vi "Teleop.vi"(10 "Match Info":T1={"Autonomous Elapsed Seconds"=0.0, "TeleOp Elapsed Seconds"=0.0, "Disabled Elapsed Seconds"=0.0, "Visited Autonomous"=FALSE, "Visited TeleOp"=FALSE, "Visited Disabled"=FALSE, "Autonomous Settings"={"Autonomous Style"=enum."Independent", "VI Refnum"=refnum}}, 11 "Call Context":T2) -> ()   [LabVIEW 2012]
doc: "This VI is called for each TeleOp packet received from the DS where the robot is not disabled. It is often used to read from the joysticks and update I/O or to update setpoints for timed control loops. It should complete and return within 20 milliseconds or it may miss DS packets."
uses:
  <vilib>/Rock Robotics/WPI/DriverStation/WPI_DriverStationDerivedRobotMode.ctl
  <vilib>/Rock Robotics/WPI/DriverStation/WPI_DriverStationMatch Info.ctl
  <vilib>/Rock Robotics/WPI/Relay/WPI_RelayValue.ctl
  Robot Global Data.vi
  <vilib>/Rock Robotics/WPI/Joystick/WPI_JoystickGetSetRefNum.vi
panel:
  in  "Ext Const":dbl=0.5
  in  "Dep Const":dbl=1.0
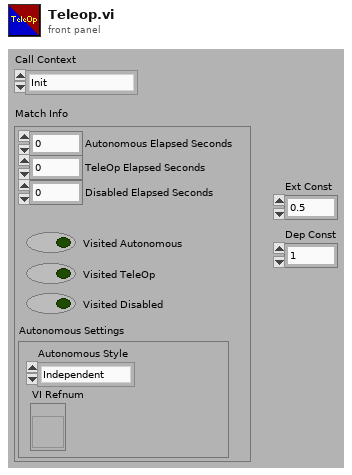
[diagram p1: front panel]
types:
  T1 = typedef "WPI_DriverStationMatch Info.ctl" = cluster{"Autonomous Elapsed Seconds":dbl, "TeleOp Elapsed Seconds":dbl, "Disabled Elapsed Seconds":dbl, "Visited Autonomous":bool, "Visited TeleOp":bool, "Visited Disabled":bool, "Autonomous Settings":cluster{"Autonomous Style":enum16{"Iterative", "Independent"}, "VI Refnum":refnum<vi>}}
  T2 = typedef "WPI_DriverStationDerivedRobotMode.ctl" = enum16{"Init", "Execute", "Stop"}
  T3 = typedef "WPI_RelayValue.ctl" = enum16{"Off", "On", "Forward", "Reverse"}
  T4 = cluster{"Driver Station Digital Input (1-8)[0]":bool, "Driver Station Digital Input (1-8)[1]":bool, "Driver Station Digital Input (1-8)[2]":bool, "Driver Station Digital Input (1-8)[3]":bool, "Driver Station Digital Input (1-8)[4]":bool, "Driver Station Digital Input (1-8)[5]":bool, "Driver Station Digital Input (1-8)[6]":bool, "Driver Station Digital Input (1-8)[7]":bool, "Driver Station Digital Input (1-8)[8]":bool}
  T5 = cluster{"Right Servo High":dbl, "Right Servo Mid":dbl, "Right Servo Low":dbl, "Left Servo High":dbl, "Left Servo Mid":dbl, "Left Servo Low":dbl}
  T6 = typedef "WPI_DigitalInputDevRef.ctl" = cluster{"DevStatus":errorcluster, "DIO Channel":T7, "Digital Module":T8}
  T7 = typedef "FPGA_DIOChannel.ctl" = enum8{"DIO 1", "DIO 2", "DIO 3", "DIO 4", "DIO 5", "DIO 6", "DIO 7", "DIO 8", "DIO 9", "DIO 10", "DIO 11", "DIO 12", "DIO 13", "DIO 14", "Invalid"}
  T8 = typedef "FPGA_TypedefDigitalModule.ctl" = enum16{"Digital Module 1", "Digital Module 2"}
  T9 = typedef "WPI_JoystickDevRef.ctl" = cluster{"Device":T10}
  T10 = typedef "WPI_JoystickDeviceEnum.ctl" = enum16{"USB 1", "USB 2", "USB 3", "USB 4", "Kinect 1", "Kinect 2"}
  T11 = cluster{"axis 1 (x)":dbl, "axis 2 (y)":dbl, "axis 3 (throttle)":dbl, "axis 4":dbl, "axis 5":dbl, "axis 6":dbl}
  T12 = typedef "WPI_RelayDevRef.ctl" = cluster{"DevStatus":errorcluster, "Relay Channel":T13, "Digital Module":T8, "Relay Direction":T14}
  T13 = typedef "FPGA_DIORelayChannel.ctl" = enum8{"Relay 1", "Relay 2", "Relay 3", "Relay 4", "Relay 5", "Relay 6", "Relay 7", "Relay 8", "Invalid"}
  T14 = typedef "WPI_RelayDirection.ctl" = enum16{"Both directions", "Forward only", "Reverse only"}
  T15 = typedef "WPI_ServoDeviceRef.ctl" = cluster{"DeviceStatus":errorcluster, "Digital Module":T8, "PWM Channel":T16, "DeadBand":T17}
  T16 = typedef "FPGA_DIOPWMChannel.ctl" = enum8{"PWM 1", "PWM 2", "PWM 3", "PWM 4", "PWM 5", "PWM 6", "PWM 7", "PWM 8", "PWM 9", "PWM 10", "Invalid"}
  T17 = typedef "WPI_PWMDeadband.ctl" = cluster{"Name":string, "maxPositivePwm":i32, "minPositivePwm":i32, "centerPwm":i32, "maxNegativePwm":i32, "minNegativePwm":i32, "angularRange":u16}
  T18 = typedef "WPI_MotorControlDeviceRef.ctl" = cluster{"DeviceStatus":errorcluster, "Type":enum16{"PWM", "CAN"}, "PWM":cluster{"Digital Module":T8, "PWM Channel":T16, "DeadBand":T17}, "CAN":cluster{"Device Number":u8, "Control Mode":T19, "Semaphore":T20, "Max Vout":dbl}, "Invert":bool, "TransformRef":T21, "InvTransformRef":T21}
  T19 = typedef "WPI_CANJaguar_ControlMode.ctl" = enum8{"Percent VBus", "Current", "Speed", "Position", "Voltage"}
  T20 = typedef "Semaphore RefNum" = refnum<k1>
  T21 = typedef "WPI_PWMTransform_ConPane.ctl" = refnum<vi>
  T22 = typedef "WPI_JoystickButtonState.ctl" = cluster{"Button 1":bool, "Button 2":bool, "Button 3":bool, "Button 4":bool, "Button 5":bool, "Button 6":bool, "Button 7":bool, "Button 8":bool, "Button 9":bool, "Button 10":bool, "Button 11":bool, "Button 12":bool}
  T23 = cluster{"FlipperLeftUp":dbl, "FlipperLeftDown":dbl, "FlipperRightUp":dbl, "FlipperRightDown":dbl, "KickerLeftBack":dbl, "KickerLeftForward":dbl, "KickerRightBack":dbl, "KickerRightForward":dbl}
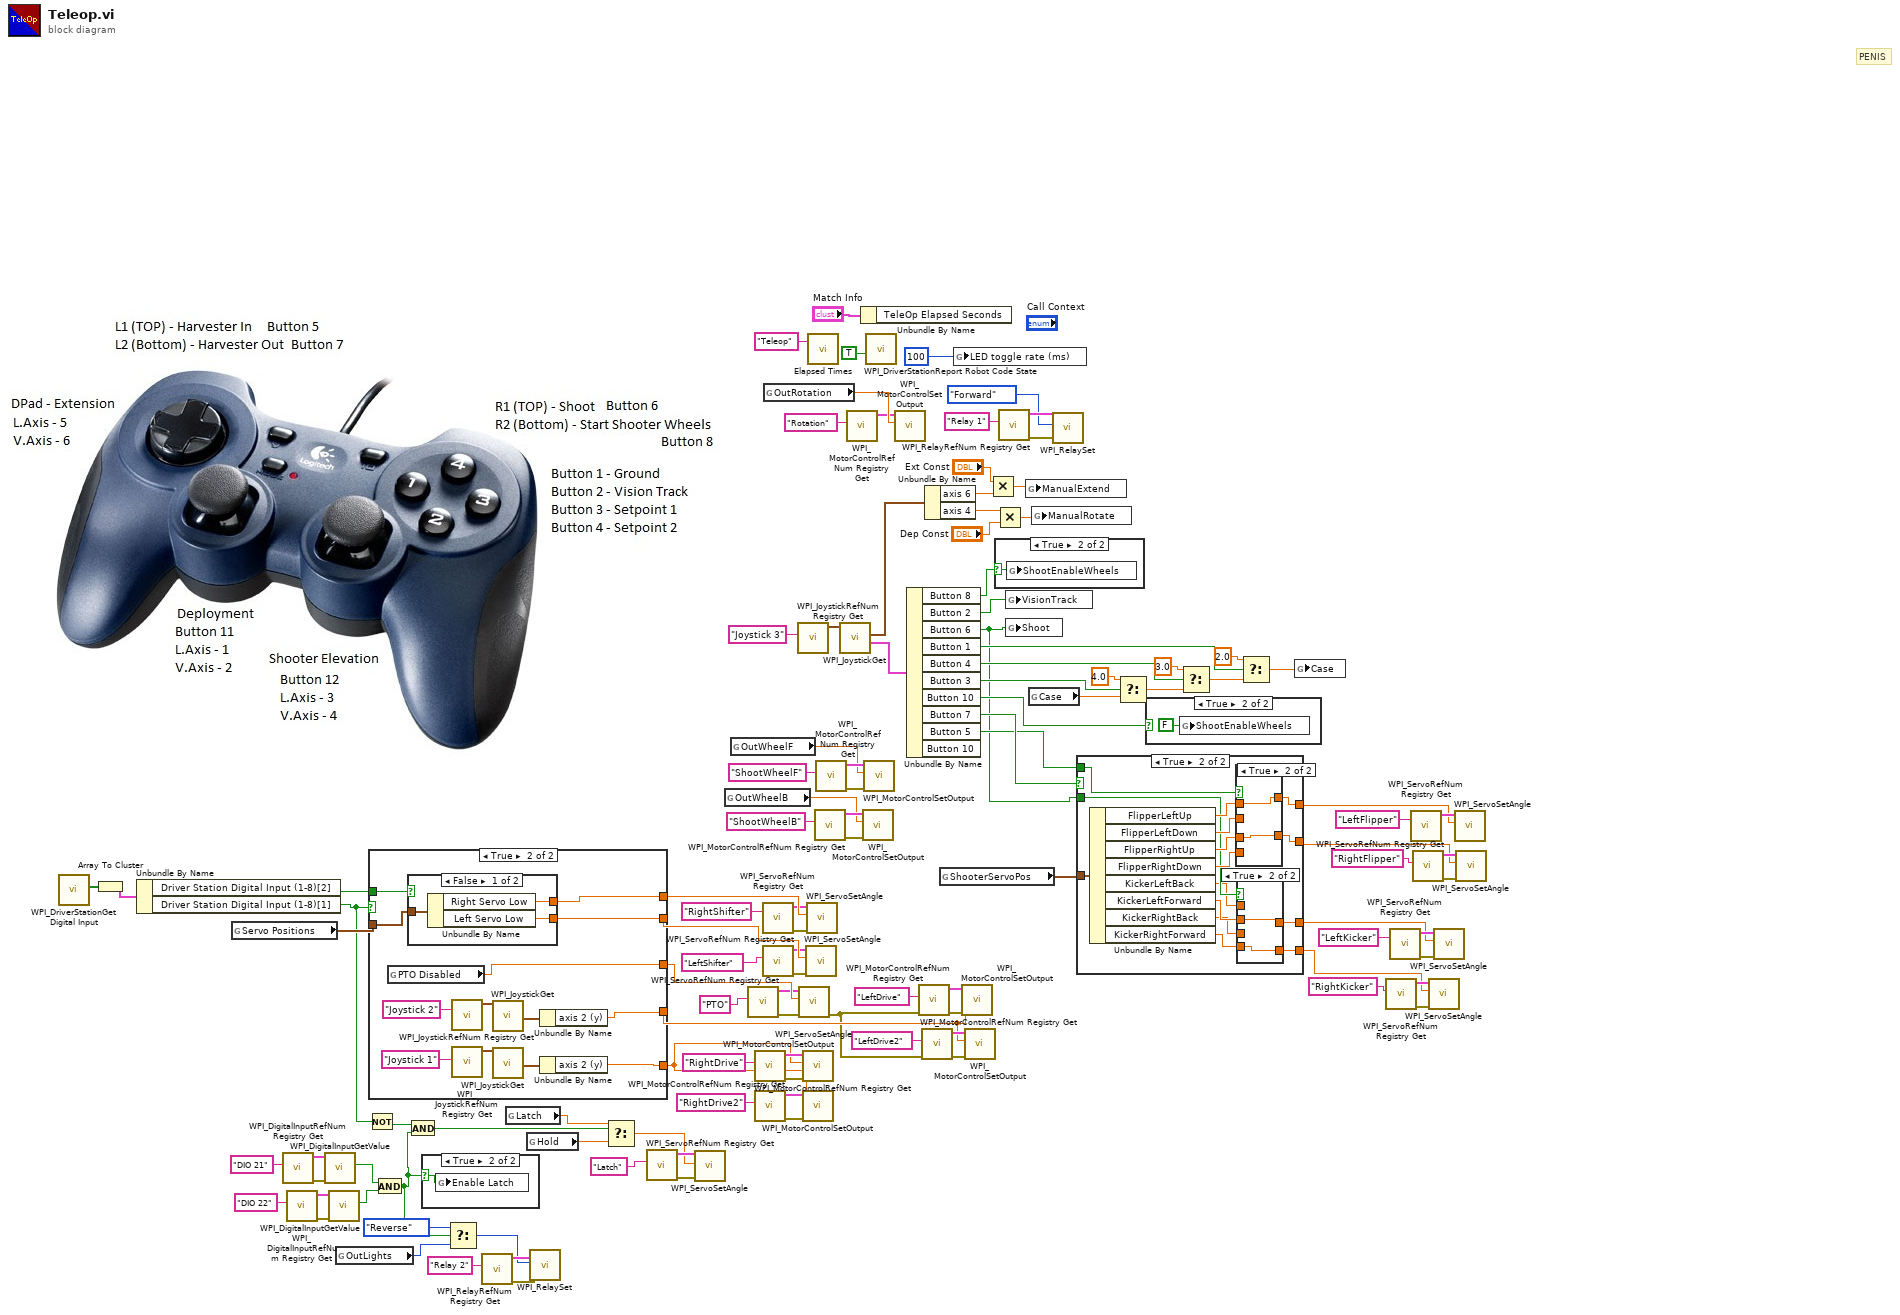
[diagram p0: block diagram]
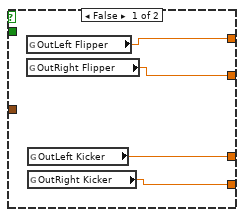
[diagram p2: hidden frame]
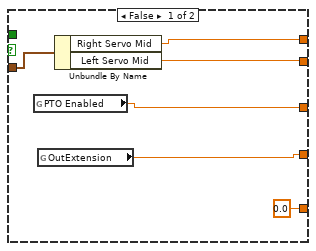
[diagram p6: hidden frame]
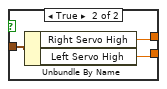
[diagram p7: hidden frame]
diagram:
  # "PENIS"
  n1 = call <vilib>:"WPI_DriverStationGet Digital Input.vi"() -> ("Driver Station Digital Input (1-8)"=w84:bool[])  [unwired: 11 in]
  n2 = Array To Cluster(array=w84) -> (cluster=w83:T4)
  n3 = Unbundle By Name(w83) -> ("Driver Station Digital Input (1-8)[2]"=w82:bool, "Driver Station Digital Input (1-8)[1]"=w35:bool)
  n4 = global read "Robot Global Data.vi" "Servo Positions"() -> (w81:T5)
  n5 = call <vilib>:"WPI_DigitalInputRefNum Registry Get.vi"("refnum name"="DIO 21") -> ("error out"=w49:errorcluster, "DigitalInputDevRef"=w42:T6)  [unwired: 9 in]
  n6 = call <vilib>:"WPI_DigitalInputRefNum Registry Get.vi"("refnum name"="DIO 22") -> ("error out"=w46:errorcluster, "DigitalInputDevRef"=w43:T6)  [unwired: 9 in]
  n7 = call <vilib>:"WPI_DigitalInputGetValue.vi"("error in (no error)"=w49, "DigitalInputDevRef"=w42) -> ("Value"=w44:bool)  [unwired: 7 in, 2 out]
  n8 = call <vilib>:"WPI_DigitalInputGetValue.vi"("error in (no error)"=w46, "DigitalInputDevRef"=w43) -> ("Value"=w45:bool)  [unwired: 7 in, 2 out]
  n9 = global read "Robot Global Data.vi" "OutLights"() -> (w41:T3)
  n10 = Not(x=w35) -> (.not. x?=w33:bool)
  n11 = case shown="True" w35 {
    tunnel: w82 -> [_ w135]
    tunnel: w81 -> [w122 w134]
    tunnel: [w121 w133] -> w80
    tunnel: [w120 w132] -> w79
    tunnel: [w119 w131] -> w72
    tunnel: [w117 w124] -> w71
    tunnel: [0.0 w123] -> w70
    frame False {
      n12 = global read "Robot Global Data.vi" "PTO Enabled"() -> (w119:dbl)
      n13 = global read "Robot Global Data.vi" "OutExtension"() -> (w117:dbl)
      n14 = Unbundle By Name(w122) -> ("Right Servo Mid"=w121:dbl, "Left Servo Mid"=w120:dbl)
    }
    frame True {
      n15 = global read "Robot Global Data.vi" "PTO Disabled"() -> (w131:dbl)
      n16 = case shown="False" w135 {
        tunnel: w134 -> [w138 w141]
        tunnel: [w137 w140] -> w133
        tunnel: [w136 w139] -> w132
        frame False {
          n17 = Unbundle By Name(w138) -> ("Right Servo Low"=w137:dbl, "Left Servo Low"=w136:dbl)
        }
        frame True {
          n18 = Unbundle By Name(w141) -> ("Right Servo High"=w140:dbl, "Left Servo High"=w139:dbl)
        }
      }
      n19 = call <vilib>:"WPI_JoystickRefNum Registry Get.vi"("refnum name"="Joystick 2") -> ("JoystickDevRef"=w125:T9)  [unwired: 1 in, 9 out]
      n20 = call <vilib>:"WPI_JoystickRefNum Registry Get.vi"("refnum name"="Joystick 1") -> ("JoystickDevRef"=w129:T9)  [unwired: 1 in, 9 out]
      n21 = call <vilib>:"WPI_JoystickGet.vi"("JoystickDevRef"=w125) -> ("Axes"=w127:T11)  [unwired: 1 in, 5 out]
      n22 = call <vilib>:"WPI_JoystickGet.vi"("JoystickDevRef"=w129) -> ("Axes"=w130:T11)  [unwired: 1 in, 5 out]
      n23 = Unbundle By Name(w127) -> ("axis 2 (y)"=w124:dbl)
      n24 = Unbundle By Name(w130) -> ("axis 2 (y)"=w123:dbl)
    }
  }
  n25 = And(x=w44, y=w45) -> (x .and. y?=w34:bool)
  n26 = And(x=w33, y=w34) -> (x .and. y?=w32:bool)
  n27 = case shown="True" w34 {
    selector: w34 -> [_ w142]
    frame False {
    }
    frame True {
      n28 = global write "Robot Global Data.vi" "Enable Latch"(w142) -> ()
    }
  }
  n29 = Select(t=WPI_RelayValue."Reverse" ("RelayValue"), s=w34, f=w41) -> (s? t:f=w39:T3)
  n30 = call <vilib>:"WPI_RelayRefNum Registry Get.vi"("refnum name"="Relay 2") -> ("error out"=w55:errorcluster, "RelayDevRef"=w53:T12)  [unwired: 9 in]
  n31 = global read "Robot Global Data.vi" "Latch"() -> (w2:dbl)
  n32 = global read "Robot Global Data.vi" "Hold"() -> (w1:dbl)
  n33 = call <vilib>:"WPI_RelaySet.vi"("error in (no error)"=w55, "RelayValue"=w39, "RelayDevRef"=w53) -> ()  [unwired: 7 in, 2 out]
  n34 = Select(t=w2, s=w32, f=w1) -> (s? t:f=w31:dbl)
  n35 = call <vilib>:"WPI_ServoRefNum Registry Get.vi"("refnum name"="Latch") -> ("error out"=w38:errorcluster, "ServoDeviceRef"=w36:T15)  [unwired: 9 in]
  n36 = call <vilib>:"WPI_ServoSetAngle.vi"("error in (no error)"=w38, "Angle"=w31, "ServoDeviceRef"=w36) -> ()  [unwired: 7 in, 2 out]
  n37 = global read "Robot Global Data.vi" "OutWheelB"() -> (w23:dbl)
  n38 = global read "Robot Global Data.vi" "OutWheelF"() -> (w24:dbl)
  n39 = call <vilib>:"WPI_ServoRefNum Registry Get.vi"("refnum name"="PTO") -> ("error out"=w65:errorcluster, "ServoDeviceRef"=w66:T15)  [unwired: 9 in]
  n40 = call <vilib>:"WPI_MotorControlRefNum Registry Get.vi"("refnum name"="RightDrive") -> ("error out"=w94:errorcluster, "MotorControlDevRef"=w96:T18)  [unwired: 9 in]
  n41 = call <vilib>:"WPI_MotorControlRefNum Registry Get.vi"("refnum name"="RightDrive2") -> ("error out"=w87:errorcluster, "MotorControlDevRef"=w85:T18)  [unwired: 9 in]
  n42 = call <vilib>:"WPI_ServoRefNum Registry Get.vi"("refnum name"="RightShifter") -> ("error out"=w75:errorcluster, "ServoDeviceRef"=w76:T15)  [unwired: 9 in]
  n43 = call <vilib>:"WPI_ServoRefNum Registry Get.vi"("refnum name"="LeftShifter") -> ("error out"=w77:errorcluster, "ServoDeviceRef"=w78:T15)  [unwired: 9 in]
  n44 = global read "Robot Global Data.vi" "OutRotation"() -> (w69:dbl)
  n45 = call <vilib>:"WPI_JoystickRefNum Registry Get.vi"("refnum name"="Joystick 3") -> ("JoystickDevRef"=w113:T9)  [unwired: 9 in, 1 out]
  n46 = call <vilib>:"WPI_ServoSetAngle.vi"("error in (no error)"=w65, "Angle"=w72, "ServoDeviceRef"=w66) -> ("error out"=w61:errorcluster)  [unwired: 7 in, 1 out]
  n47 = call <vilib>:"WPI_MotorControlSetOutput.vi"("error in (no error)"=w94, "Output"=w70, "MotorControlDevRef"=w96) -> ()  [unwired: 6 in, 3 out]
  n48 = call <vilib>:"WPI_MotorControlSetOutput.vi"("error in (no error)"=w87, "Output"=w70, "MotorControlDevRef"=w85) -> ()  [unwired: 6 in, 3 out]
  n49 = call <vilib>:"WPI_ServoSetAngle.vi"("error in (no error)"=w77, "Angle"=w79, "ServoDeviceRef"=w78) -> ()  [unwired: 7 in, 2 out]
  n50 = call <vilib>:"WPI_ServoSetAngle.vi"("error in (no error)"=w75, "Angle"=w80, "ServoDeviceRef"=w76) -> ()  [unwired: 7 in, 2 out]
  n51 = call "Elapsed Times.vi"("Call Name"="Teleop") -> ()  [unwired: 2 in, 1 out]
  n52 = call <vilib>:"WPI_MotorControlRefNum Registry Get.vi"("refnum name"="ShootWheelB") -> ("error out"=w26:errorcluster, "MotorControlDevRef"=w27:T18)  [unwired: 9 in]
  n53 = call <vilib>:"WPI_MotorControlRefNum Registry Get.vi"("refnum name"="ShootWheelF") -> ("error out"=w28:errorcluster, "MotorControlDevRef"=w25:T18)  [unwired: 9 in]
  n54 = call <vilib>:"WPI_JoystickGet.vi"("JoystickDevRef"=w113) -> ("Buttons"=w111:T22, "Axes"=w110:T11)  [unwired: 4 in, 1 out]
  n55 = call <vilib>:"WPI_MotorControlRefNum Registry Get.vi"("refnum name"="Rotation") -> ("MotorControlDevRef"=w67:T18)  [unwired: 9 in, 1 out]
  n56 = Unbundle By Name("Match Info") -> ()  [unwired: 1 out]
  n57 = call <vilib>:"WPI_MotorControlSetOutput.vi"("error in (no error)"=w26, "Output"=w23, "MotorControlDevRef"=w27) -> ()  [unwired: 6 in, 3 out]
  n58 = call <vilib>:"WPI_MotorControlSetOutput.vi"("error in (no error)"=w28, "Output"=w24, "MotorControlDevRef"=w25) -> ()  [unwired: 6 in, 3 out]
  n59 = call <vilib>:"WPI_DriverStationReport Robot Code State.vi"("TeleOp"=TRUE ("Autonomous")) -> ()  [unwired: 10 in, 1 out]
  n60 = call <vilib>:"WPI_MotorControlSetOutput.vi"("Output"=w69, "MotorControlDevRef"=w67) -> ()  [unwired: 7 in, 3 out]
  n61 = Unbundle By Name(w111) -> ("Button 8"=w98:bool, "Button 2"=w109:bool, "Button 6"=w4:bool, "Button 1"=w108:bool, "Button 4"=w106:bool, "Button 3"=w105:bool, "Button 10"=w22:bool, "Button 7"=w21:bool, "Button 5"=w20:bool)  [unwired: 1 out]
  n62 = call <vilib>:"WPI_MotorControlRefNum Registry Get.vi"("error in (no error)"=w61, "refnum name"="LeftDrive") -> ("error out"=w89:errorcluster, "MotorControlDevRef"=w92:T18)  [unwired: 8 in]
  n63 = call <vilib>:"WPI_MotorControlRefNum Registry Get.vi"("error in (no error)"=w61, "refnum name"="LeftDrive2") -> ("error out"=w88:errorcluster, "MotorControlDevRef"=w90:T18)  [unwired: 8 in]
  n64 = Unbundle By Name(w110) -> ("axis 6"=w52:dbl, "axis 4"=w62:dbl)
  n65 = global read "Robot Global Data.vi" "ShooterServoPos"() -> (w5:T23)
  n66 = global write "Robot Global Data.vi" "LED toggle rate (ms)"(u32 100 ("LED ms toggle rate")) -> ()
  n67 = call <vilib>:"WPI_MotorControlSetOutput.vi"("error in (no error)"=w89, "Output"=w71, "MotorControlDevRef"=w92) -> ()  [unwired: 6 in, 3 out]
  n68 = call <vilib>:"WPI_MotorControlSetOutput.vi"("error in (no error)"=w88, "Output"=w71, "MotorControlDevRef"=w90) -> ()  [unwired: 6 in, 3 out]
  n69 = Multiply(x="Ext Const", y=w52) -> (x*y=w50:dbl)
  n70 = Multiply(x=w62, y="Dep Const") -> (x*y=w60:dbl)
  n71 = case shown="True" w98 {
    selector: w98 -> [_ w143]
    frame False {
    }
    frame True {
      n72 = global write "Robot Global Data.vi" "ShootEnableWheels"(w143) -> ()
    }
  }
  n73 = call <vilib>:"WPI_RelayRefNum Registry Get.vi"("refnum name"="Relay 1") -> ("error out"=w57:errorcluster, "RelayDevRef"=w59:T12)  [unwired: 9 in]
  n74 = global write "Robot Global Data.vi" "VisionTrack"(w109) -> ()
  n75 = global write "Robot Global Data.vi" "Shoot"(w4) -> ()
  n76 = global write "Robot Global Data.vi" "ManualExtend"(w50) -> ()
  n77 = global read "Robot Global Data.vi" "Case"() -> (w100:dbl)
  n78 = global write "Robot Global Data.vi" "ManualRotate"(w60) -> ()
  n79 = call <vilib>:"WPI_RelaySet.vi"("error in (no error)"=w57, "RelayValue"=WPI_RelayValue."Forward", "RelayDevRef"=w59) -> ()  [unwired: 7 in, 2 out]
  n80 = case shown="True" w21 {
    tunnel: w20 -> [_ w148]
    tunnel: [w147 w161] -> w8
    tunnel: [w146 w159] -> w7
    tunnel: [w145 w150] -> w6
    tunnel: [w144 w149] -> w3
    tunnel: w5 -> [_ w162]
    tunnel: w4 -> [_ w155]
    frame False {
      n81 = global read "Robot Global Data.vi" "OutLeft Flipper"() -> (w147:dbl)
      n82 = global read "Robot Global Data.vi" "OutRight Flipper"() -> (w146:dbl)
      n83 = global read "Robot Global Data.vi" "OutLeft Kicker"() -> (w145:dbl)
      n84 = global read "Robot Global Data.vi" "OutRight Kicker"() -> (w144:dbl)
    }
    frame True {
      n85 = Unbundle By Name(w162) -> ("FlipperLeftUp"=w160:dbl, "FlipperLeftDown"=w157:dbl, "FlipperRightUp"=w158:dbl, "FlipperRightDown"=w156:dbl, "KickerLeftBack"=w154:dbl, "KickerLeftForward"=w153:dbl, "KickerRightBack"=w152:dbl, "KickerRightForward"=w151:dbl)
      n86 = case shown="True" w148 {
        tunnel: [w168 w170] -> w161
        tunnel: w160 -> [_ w170]
        tunnel: [w167 w169] -> w159
        tunnel: w158 -> [_ w169]
        tunnel: w157 -> [w168 _]
        tunnel: w156 -> [w167 _]
        frame False {
        }
        frame True {
        }
      }
      n87 = case shown="True" w155 {
        tunnel: w154 -> [w164 _]
        tunnel: w153 -> [_ w165]
        tunnel: w152 -> [w163 _]
        tunnel: w151 -> [_ w166]
        tunnel: [w164 w165] -> w150
        tunnel: [w163 w166] -> w149
        frame False {
        }
        frame True {
        }
      }
    }
  }
  n88 = Select(t=4.0, s=w105, f=w100) -> (s? t:f=w104:dbl)
  n89 = case shown="True" w22 {
    frame False {
    }
    frame True {
      n90 = global write "Robot Global Data.vi" "ShootEnableWheels"(FALSE ("ShootStartWheels")) -> ()
    }
  }
  n91 = Select(t=3.0, s=w106, f=w104) -> (s? t:f=w102:dbl)
  n92 = Select(t=2.0, s=w108, f=w102) -> (s? t:f=w99:dbl)
  n93 = global write "Robot Global Data.vi" "Case"(w99) -> ()
  n94 = call <vilib>:"WPI_ServoRefNum Registry Get.vi"("refnum name"="RightKicker") -> ("error out"=w17:errorcluster, "ServoDeviceRef"=w15:T15)  [unwired: 9 in]
  n95 = call <vilib>:"WPI_ServoRefNum Registry Get.vi"("refnum name"="LeftKicker") -> ("error out"=w9:errorcluster, "ServoDeviceRef"=w10:T15)  [unwired: 9 in]
  n96 = call <vilib>:"WPI_ServoRefNum Registry Get.vi"("refnum name"="LeftFlipper") -> ("ServoDeviceRef"=w11:T15)  [unwired: 9 in, 1 out]
  n97 = call <vilib>:"WPI_ServoRefNum Registry Get.vi"("refnum name"="RightFlipper") -> ("error out"=w19:errorcluster, "ServoDeviceRef"=w12:T15)  [unwired: 9 in]
  n98 = call <vilib>:"WPI_ServoSetAngle.vi"("error in (no error)"=w17, "Angle"=w3, "ServoDeviceRef"=w15) -> ()  [unwired: 7 in, 2 out]
  n99 = call <vilib>:"WPI_ServoSetAngle.vi"("error in (no error)"=w9, "Angle"=w6, "ServoDeviceRef"=w10) -> ()  [unwired: 7 in, 2 out]
  n100 = call <vilib>:"WPI_ServoSetAngle.vi"("Angle"=w8, "ServoDeviceRef"=w11) -> ()  [unwired: 8 in, 2 out]
  n101 = call <vilib>:"WPI_ServoSetAngle.vi"("error in (no error)"=w19, "Angle"=w7, "ServoDeviceRef"=w12) -> ()  [unwired: 7 in, 2 out]
